vi "DAQ_Mea_sub.vi"(2 "Sampling Num":i32=300, 3 "speed":dbl=20000.0) -> (0 "vol_out":dbl=1.4632930663926527, 1 "웨이브폼 그래프 2":dbl[](graph)=[1.1723181982524693, 1.1684486800804734, 1.1697385194711387, 1.1697385194711387, 1.1684486800804734, 1.161999483127147, 1.161999483127147, 1.161999483127147, 1.1607096437364817, 1.1568401255644858, 1.1568401255644858, 1.1503909286111593, 1.1478112498298287, 1.1542604467831552, 1.1478112498298287, 1.1452315710484982, 1.1465214104391634, 1.1439417316578329, 1.1387823740951717, 1.1387823740951717, 1.1413620528765023, 1.1426518922671676, 1.1387823740951717, 1.1426518922671676, 1.1374925347045064, 1.1413620528765023, 1.140072213485837, 1.1413620528765023, 1.140072213485837, 1.1478112498298287, 1.158129964955151, 1.1555502861738205, 1.1594198043458164, 1.1632893225178123, 1.1645791619084775, 1.1697385194711387, 1.1697385194711387, 1.1684486800804734, 1.1736080376431346, 1.1761877164244652, 1.1774775558151305, 1.1748978770337999, 1.1826369133777916, 1.1826369133777916, 1.183926752768457, 1.189086110331118, 1.1916657891124487, 1.192955628503114, 1.2032743436284363, 1.201984504237771, 1.211013379972428, 1.2123032193630934, 1.214882898144424, 1.2226219344884157, 1.223911773879081, 1.2316508102230728, 1.2342304890044034, 1.2381000071763992, 1.2471288829110563, 1.2484187223017216, 1.2509984010830522, 1.2574475980363786, 1.2651866343803704, 1.2703459919430315, 1.2664764737710357, 1.276795188896358, 1.2819545464590192, 1.2819545464590192, 1.2871139040216804, 1.298722458537668, 1.2974326191470027, 1.3013021373189986, 1.3064614948816597, 1.3129106918349862, 1.311620852444321, 1.320649728178978, 1.3258090857416391, 1.329678603913635, 1.3283887645229697, 1.3361278008669615, 1.3477363553829491, 1.3438668372109532, 1.3528957129456103, 1.3619245886802673, 1.3683737856335938, 1.3683737856335938, 1.3748229825869203, 1.3812721795402467, 1.3890112158842385, 1.386431537102908, 1.3967502522282302, 1.3993299310095608, 1.4083588067442179, 1.4070689673535526, 1.4148080036975443, 1.4160978430882096, 1.4212572006508708, 1.4186775218695402, 1.4289962369948626, 1.4367352733388543, 1.444474309682846, 1.444474309682846, 1.4496336672455072, 1.4560828641988337, 1.457372703589499, 1.4651117399334908, 1.4728507762774825, 1.4767202944494784, 1.4818796520121396, 1.492198367137462, 1.492198367137462, 1.501227242872119, 1.5050967610441148, 1.5128357973881066, 1.5167053155601025, 1.52831387007609, 1.5257341912947595, 1.5347630670294166, 1.545081782154739, 1.5489513003267348, 1.5528208184987307, 1.5605598548427224, 1.5657192124053836, 1.5799074457027018, 1.5799074457027018, 1.5863566426560283, 1.5915160002186894, 1.5953855183906853, 1.6057042335160077, 1.6121534304693341, 1.6121534304693341, 1.6121534304693341, 1.625051824375987, 1.628921342547983, 1.6315010213293135, 1.634080700110644, 1.6443994152359664, 1.6443994152359664, 1.6495587727986276, 1.646979094017297, 1.656007969751954, 1.6572978091426194, 1.65987748792395, 1.6624571667052805, 1.6663266848772764, 1.6650368454866111, 1.6663266848772764, 1.6740657212212682, 1.6727758818306029, 1.6766454000025988, 1.677935239393264, 1.677935239393264, 1.68180475756526, 1.6843844363465905, 1.6856742757372558, 1.6947031514719129, 1.6895437939092517, 1.6882539545185864, 1.6959929908625782, 1.7011523484252393, 1.6959929908625782, 1.7011523484252393, 1.699862509034574, 1.7063117059879005, 1.70373202720657, 1.7011523484252393, 1.7024421878159046, 1.708891384769231, 1.7063117059879005, 1.7011523484252393, 1.712760902941227, 1.7050218665972352, 1.7050218665972352, 1.712760902941227, 1.7101812241598964, 1.7114710635505617, 1.712760902941227, 1.7179202605038881, 1.712760902941227, 1.7153405817225575, 1.7192100998945534, 1.7166304211132228, 1.7179202605038881, 1.7166304211132228, 1.7204999392852187, 1.7204999392852187, 1.7192100998945534, 1.7153405817225575, 1.7179202605038881, 1.7230796180665493, 1.7192100998945534, 1.7179202605038881, 1.7192100998945534, 1.7140507423318923, 1.7101812241598964, 1.7076015453785658, 1.7050218665972352, 1.6985726696439087, 1.7011523484252393, 1.6985726696439087, 1.6921234726905823, 1.6895437939092517, 1.6934133120812476, 1.6934133120812476, 1.6843844363465905, 1.6895437939092517, 1.6856742757372558, 1.6856742757372558, 1.6830945969559252, 1.6843844363465905, 1.6792250787839293, 1.6792250787839293, 1.6727758818306029, 1.6766454000025988, 1.6701962030492723, 1.6714860424399376, 1.6637470060959458, 1.6611673273146152, 1.6572978091426194, 1.6495587727986276, 1.6521384515799582, 1.63795021828264, 1.63795021828264, 1.634080700110644, 1.6263416637666523, 1.628921342547983, 1.625051824375987, 1.6147331092506647, 1.6198924668133259, 1.6121534304693341, 1.6095737516880035, 1.6005448759533465, 1.5966753577813506, 1.6005448759533465, 1.5928058396093547, 1.5876464820466936, 1.585066803265363, 1.5824871244840324, 1.5799074457027018, 1.5734582487493753, 1.5695887305773795, 1.5605598548427224, 1.5592700154520571, 1.5592700154520571, 1.5528208184987307, 1.5463716215454042, 1.5425021033734083, 1.5360529064200819, 1.5347630670294166, 1.5270240306854248, 1.5205748337320983, 1.5154154761694372, 1.510256118606776, 1.501227242872119, 1.497357724700123, 1.4986475640907884, 1.4934882065281272, 1.4857491701841354, 1.4818796520121396, 1.4818796520121396, 1.475430455058813, 1.4715609368868172, 1.4625320611521602, 1.4599523823708296, 1.457372703589499, 1.4535031854175031, 1.4470539884641767, 1.4431844702921808, 1.4341555945575237, 1.4289962369948626, 1.4277063976041973, 1.4148080036975443, 1.413518164306879, 1.4083588067442179, 1.4057791279628873, 1.3967502522282302, 1.3890112158842385, 1.3812721795402467, 1.3799823401495814, 1.3683737856335938, 1.364504267461598, 1.3619245886802673, 1.3567652311176062, 1.3451566766016185, 1.342576997820288, 1.3374176402576268, 1.3283887645229697, 1.320649728178978, 1.3232294069603086, 1.3090411736629903, 1.3051716554909945, 1.3000122979283333, 1.2961427797563374, 1.285824064631015, 1.2780850282870233, 1.276795188896358, 1.2742155101150274, 1.2651866343803704, 1.2522882404737175, 1.2535780798643827])   [LabVIEW 2021]
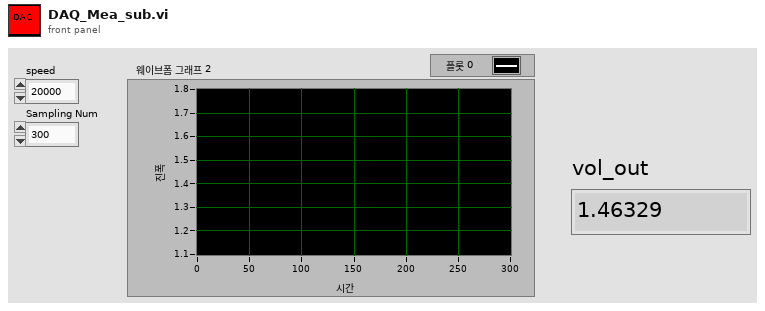
[diagram p1: front panel]
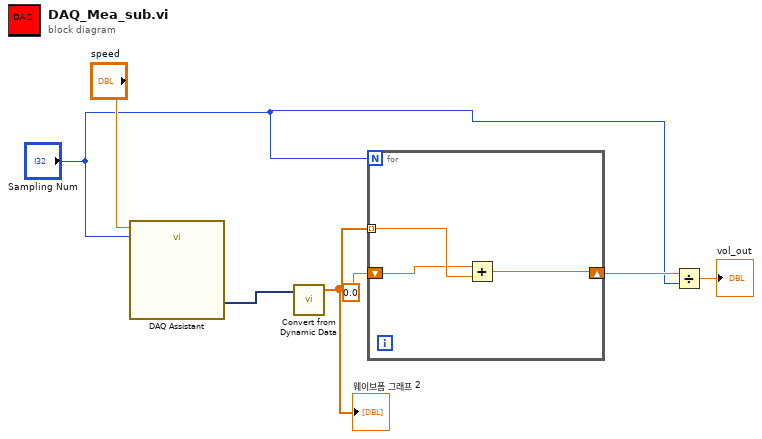
[diagram p0: block diagram]
diagram:
  n1 = call "DAQ Assistant"("rate"="speed", "number of samples"="Sampling Num") -> ("data"=w6:dynamicdata)  [unwired: 14 in, 3 out]
  n2 = call "Convert from Dynamic Data"("Dynamic Data Type"=w6) -> ("Array"=w2:dbl[])  [unwired: 3 in]
  "웨이브폼 그래프 2" <- w2
  n3 = for {
    N: "Sampling Num" -> [_]
    tunnel: w2 -> [w10] mode=indexing
    shift-right: [w9] -> w5
    shift-left: 0.0 -> [w8]
    n4 = Add(x=w8, y=w10) -> (x+y=w9:dbl)
  }
  n5 = Divide(x=w5, y="Sampling Num") -> (x/y=→"vol_out":dbl)
